vi "CMI ckd2 Panel.vi"(8 "error in":errorcluster, 11 "session in":T2) -> (0 "error out":errorcluster, 3 "session out":T2)   [LabVIEW 2020, in "AWG.lvlib"]
doc: "CMI clock divider v2 configuration panel."
uses:
  AWG.lvlib
  varilib/varilib.lvlib
  CMI ckd2 Source Mode.ctl
  CMI ckd2 Session.ctl
  CMI ckd2 Divisor Mode.ctl
panel:
  in  "div mode":T1 caption="Divisor factor setup mode"
  in  "btn test":bool
  out "error":string caption="Error"
  out "meas freq":dbl caption="Input frequency [Hz]" format="%_7p"
  out "idn string":string caption="Device identification string"
  in  "btn ok":bool
  in  "fixed fref":bool caption="Use manual reference frequency entry"
  in  "fref":dbl caption="Manual reference clock [Hz]" format="%#_8p"
  in  "Clock source":T3
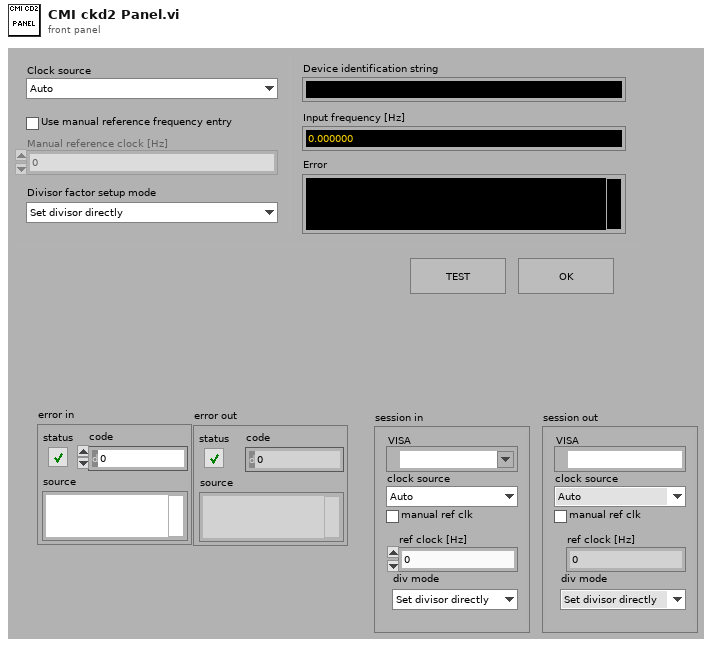
[diagram p1: front panel]
types:
  T1 = typedef "AWG.lvlib/CMI ckd2 Divisor Mode.ctl" = enum16{"Set divisor directly", "Set divisor by frequency"}
  T2 = typedef "AWG.lvlib/CMI ckd2 Session.ctl" = cluster{"VISA":refnum<visa-resource-name>, "clock source":T3, "manual ref clk":bool, "ref clock [Hz]":dbl, "div mode":T1}
  T3 = typedef "AWG.lvlib/CMI ckd2 Source Mode.ctl" = enum16{"Auto", "LF clock", "HF clock", "Internal"}
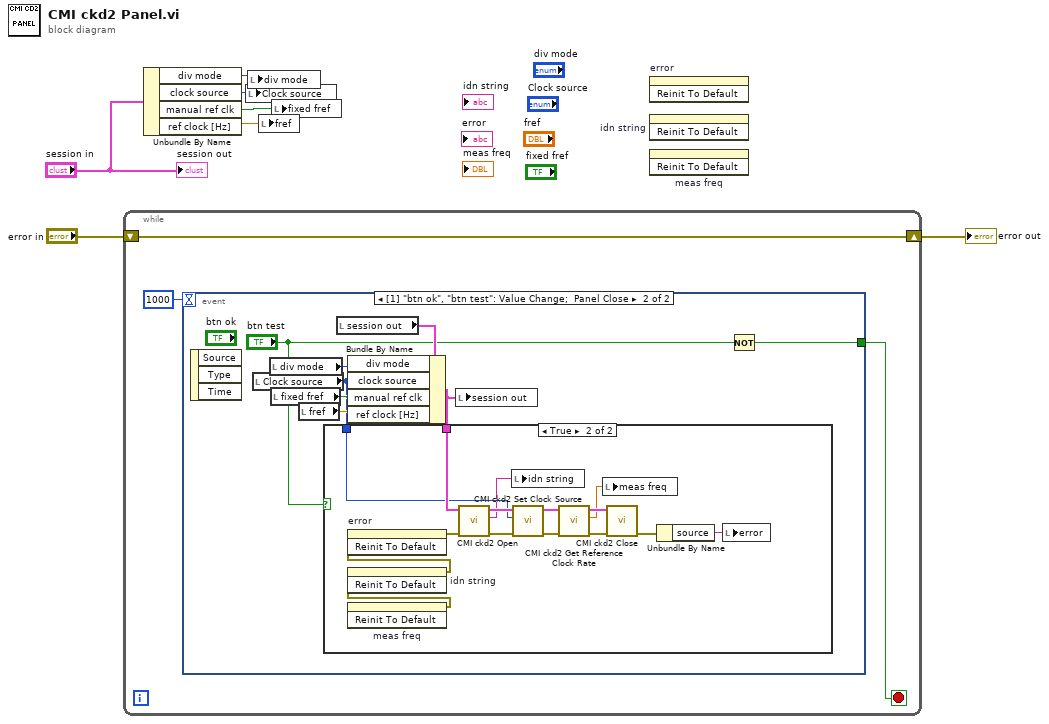
[diagram p0: block diagram]
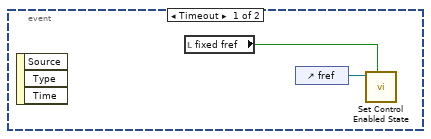
[diagram p2: hidden frame]
diagram:
  n1 = while {
    shift-right: [w9] -> w4
    shift-left: "error in" -> [w9]
    stop <- w10 stop-if-true
    n2 = event shown="[1] \"btn ok\", \"btn test\": Value Change;  Panel Close" {
      selector: _ -> [_ _]
      dyn-events: _ -> [_ _]
      timeout: 1000 -> [_ _]
      tunnel: [_ w17] -> w10
      event Timeout {
        n3 = event-data() -> ()  [unwired: 1 in, 3 out]
        n4 = local read "fixed fref"() -> (w12:bool)
        n5 = control-ref of="fref"() -> (w11:refnum<vi>)
        n6 = call "Set Control Enabled State.vi"("enabled (T)"=w12, "reference in"=w11) -> ()  [unwired: 8 in, 2 out]
      }
      event "btn ok", "btn test": Value Change; Panel Close {
        n7 = event-data() -> ()  [unwired: 1 in, 3 out]
        n8 = local read "Clock source"() -> (w14:T3)
        n9 = local read "div mode"() -> (w13:T1)
        n10 = local read "fixed fref"() -> (w19:bool)
        n11 = local read "fref"() -> (w18:dbl)
        n12 = local read "session out"() -> (w20:T2)
        n13 = Bundle By Name(cluster=w20, "div mode"=w13, "clock source"=w14, "manual ref clk"=w19, "ref clock [Hz]"=w18) -> (w15:T2)
        n14 = case shown="True" "btn test" {
          tunnel: w15 -> [_ w35]
          tunnel: w14 -> [_ w31]
          frame False {
          }
          frame True {
            n15 = invoke on="meas freq" class="DigNum (strict)" method="Reinit To Default"() -> (error out=w21:errorcluster)  [unwired: 3 in, 2 out]
            n16 = invoke on="idn string" class="Str" method="Reinit To Default"(error in=w21) -> (error out=w22:errorcluster)  [unwired: 2 in, 2 out]
            n17 = invoke on="error" class="Str" method="Reinit To Default"(error in=w22) -> (error out=w34:errorcluster)  [unwired: 2 in, 2 out]
            n18 = call "CMI ckd2 Open.vi"("error in"=w34, "session"=w35) -> ("error out"=w33:errorcluster, "read buffer"=w23:string, "session out"=w32:T2)  [unwired: 7 in]
            n19 = local write "idn string"(w23) -> ()
            n20 = call "CMI ckd2 Set Clock Source.vi"("error in"=w33, "clock source (auto)"=w31, "session"=w32) -> ("error out"=w30:errorcluster, "session out"=w29:T2)  [unwired: 7 in]
            n21 = call "CMI ckd2 Get Reference Clock Rate.vi"("error in"=w30, "session"=w29) -> ("error out"=w28:errorcluster, "clock rate [Hz]"=w26:dbl, "session out"=w27:T2)  [unwired: 7 in]
            n22 = local write "meas freq"(w26) -> ()
            n23 = call "CMI ckd2 Close.vi"("error in"=w28, "session"=w27) -> ("error out"=w25:errorcluster)  [unwired: 8 in, 1 out]
            n24 = Unbundle By Name(w25) -> ("source"=w24:string)
            n25 = local write "error"(w24) -> ()
          }
        }
        n26 = local write "session out"(w15) -> ()
        n27 = Not(x="btn test") -> (.not. x?=w17:bool)
      }
    }
  }
  "error out" <- w4
  n28 = Unbundle By Name("session in") -> ("div mode"=w1:T1, "clock source"=w7:T3, "manual ref clk"=w6:bool, "ref clock [Hz]"=w5:dbl)
  n29 = local write "Clock source"(w7) -> ()
  n30 = local write "div mode"(w1) -> ()
  n31 = local write "fref"(w5) -> ()
  n32 = local write "fixed fref"(w6) -> ()
  n33 = invoke on="error" class="Str" method="Reinit To Default"() -> ()  [unwired: 3 in, 3 out]
  n34 = invoke on="idn string" class="Str" method="Reinit To Default"() -> ()  [unwired: 3 in, 3 out]
  n35 = invoke on="meas freq" class="DigNum (strict)" method="Reinit To Default"() -> ()  [unwired: 3 in, 3 out]
  "session out" <- "session in"
